vi "AlliGator Read RecSettings.txt File.vi"(8 "Error In":errorcluster, 11 "Folder Path":path) -> (0 "Error Out":errorcluster, 1 "Metadata":T1 {"Date" format="%<%x %.3X>T"}, 3 "Settings String":string)   [LabVIEW 2021, in "AlliGator Files.lvlib"]
doc: "Tries to extract FLI dataset metadata corresponding to one of LaVision formats."
uses:
  AlliGator Files.lvlib
  AlliGator RecSettings Metadata.ctl
  AlliGator RecSettings Metadata Field.ctl
  <vilib>/Utility/error.llb/whitespace.ctl
  Time/PicoStart Date.ctl
  <vilib>/Utility/error.llb/Error Cluster From Error Code.vi
  <vilib>/ErrorRing/Error Ring.xnode
  Time/Time.lvlib
  Error/Error.lvlib
panel:
  # "see the AlliGator License on the block diagram (Ctrl+E or Window:Show Block Diagram)"
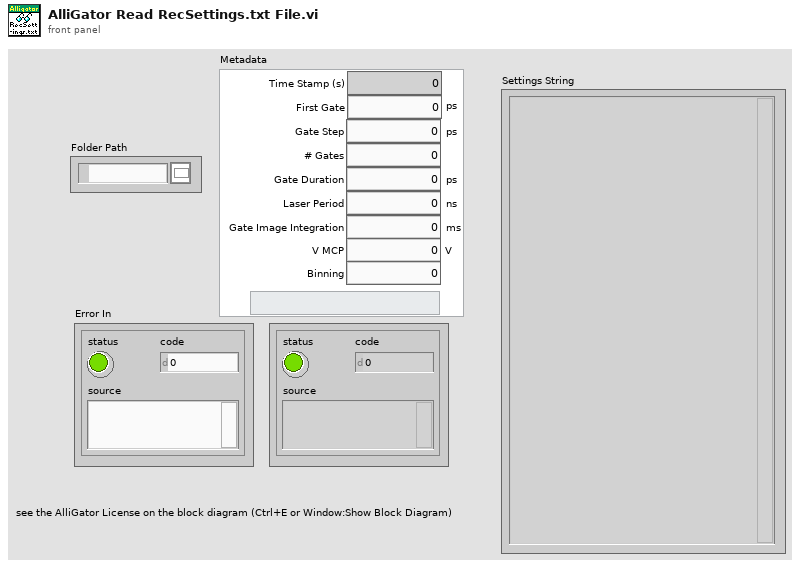
[diagram p1: front panel]
types:
  T1 = typedef "AlliGator Files.lvlib/AlliGator RecSettings Metadata.ctl" = cluster{"Time Stamp (s)":dbl, "First Gate":dbl[unit], "Gate Step":dbl[unit], "# Gates":i32, "Gate Duration":dbl[unit], "Laser Period":dbl[unit], "Gate Image Integration":dbl[unit], "Date":timestamp, "V MCP":dbl[unit], "Binning":dbl}
  T2 = typedef "Time.lvlib/PicoStart Date.ctl" = cluster{"Day in Week":string, "Month":string, "Day":i32, "Hours":i32, "Minutes":i32, "Seconds":i32, "Year":i32}
  T3 = typedef "AlliGator Files.lvlib/AlliGator RecSettings Metadata Field.ctl" = enum16{"Time", "Gate Start", "Gate Step", "# Gates", "Gate Duration", "Laser Period", "Gate Image Integration", "MCP Voltage", "Binning"}
  T4 = typedef "whitespace.ctl" = u16
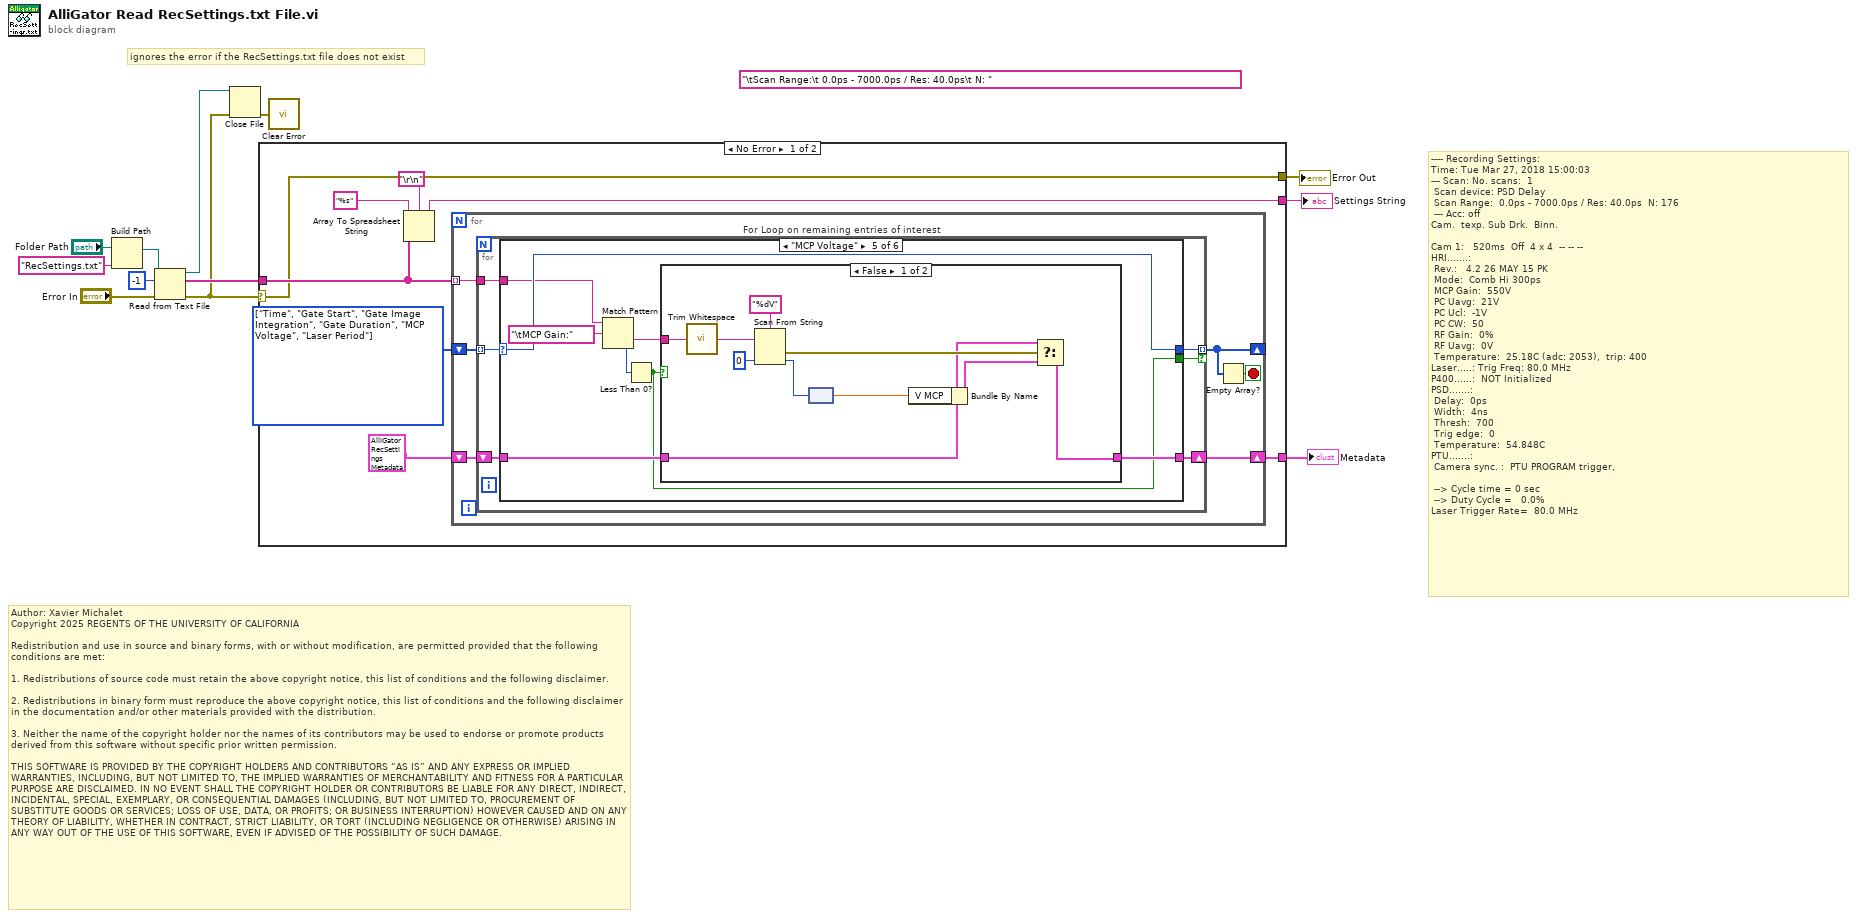
[diagram p0: block diagram]
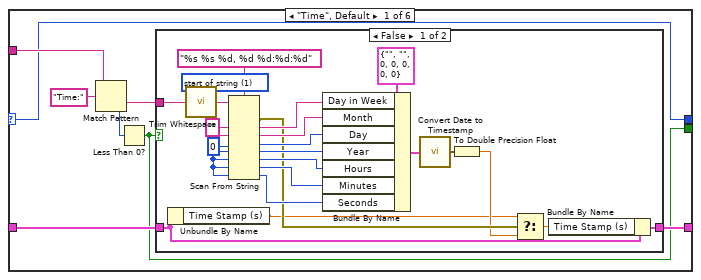
[diagram p2: hidden frame]
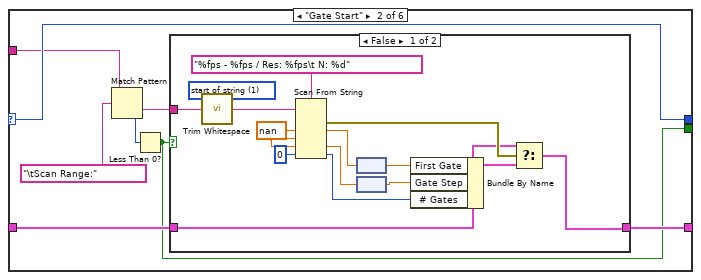
[diagram p4: hidden frame]
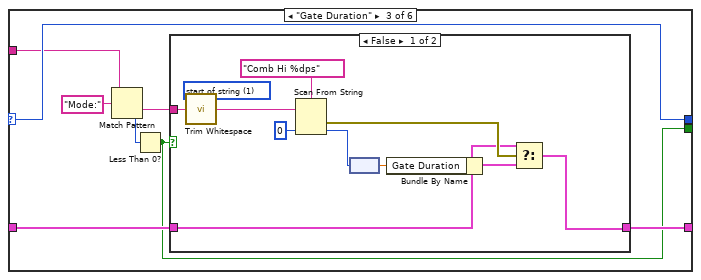
[diagram p6: hidden frame]
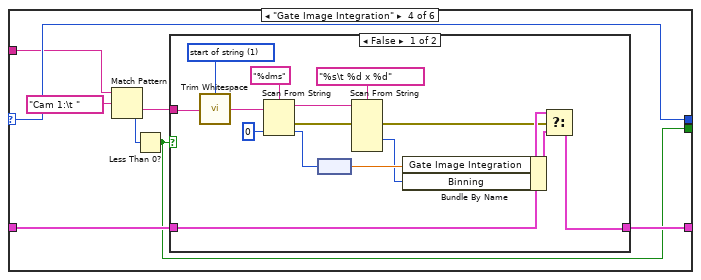
[diagram p8: hidden frame]
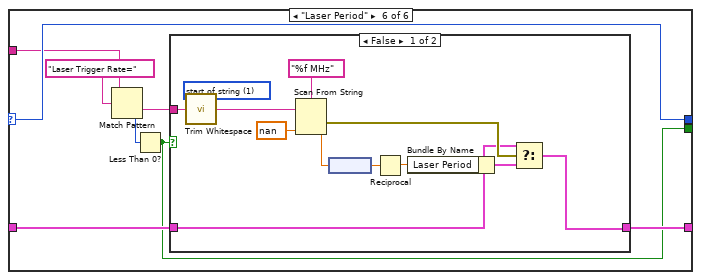
[diagram p11: hidden frame]
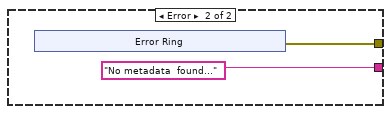
[diagram p13: hidden frame]
diagram:
  (unwired) "\tScan Range:\t 0.0ps - 7000.0ps / Res: 40.0ps\t N: "
  # "Author: Xavier Michalet\nCopyright 2025 REGENTS OF THE UNIVERSITY OF CALIFORNIA\n\nRedistribution and use in source and binary forms, with or without modification, are permitted provided that the following conditions are met:\n\n1. Redistributions of source code must retain the above copyright notice, this list of conditions and the following disclaimer.\n\n2. Redistributions in binary form must reproduce the above copyright notice, this list of conditions and the following disclaimer in the documentation and/or other materials provided with the distribution.\n\n3. Neither the name of the copyright holder nor the names of its contributors may be used to endorse or promote products derived from this software without specific prior written permission.\n\nTHIS SOFTWARE IS PROVIDED BY THE COPYRIGHT HOLDERS AND CONTRIBUTORS “AS IS” AND ANY EXPRESS OR IMPLIED WARRANTIES, INCLUDING, BUT NOT LIMITED TO, THE IMPLIED WARRANTIES OF MERCHANTABILITY AND FITNESS FOR A PARTICULAR PURPOSE ARE DISCLAIMED. IN NO EVENT SHALL THE COPYRIGHT HOLDER OR CONTRIBUTORS BE LIABLE FOR ANY DIRECT, INDIRECT, INCIDENTAL, SPECIAL, EXEMPLARY, OR CONSEQUENTIAL DAMAGES (INCLUDING, BUT NOT LIMITED TO, PROCUREMENT OF SUBSTITUTE GOODS OR SERVICES; LOSS OF USE, DATA, OR PROFITS; OR BUSINESS INTERRUPTION) HOWEVER CAUSED AND ON ANY THEORY OF LIABILITY, WHETHER IN CONTRACT, STRICT LIABILITY, OR TORT (INCLUDING NEGLIGENCE OR OTHERWISE) ARISING IN ANY WAY OUT OF THE USE OF THIS SOFTWARE, EVEN IF ADVISED OF THE POSSIBILITY OF SUCH DAMAGE."
  # "---- Recording Settings:\t\t\t\t\t\t\t\nTime:\tTue Mar 27, 2018 15:00:03\n--- Scan:\tNo. scans: \t1\n\tScan device:\tPSD Delay\n\tScan Range:\t 0.0ps - 7000.0ps / Res: 40.0ps\t N: 176\n\t--- Acc:\toff\nCam.\t texp.\tSub Drk. \tBinn.\n\nCam 1:\t  520ms\t Off\t 4 x 4\t\t--\t--\t--\nHRI.......:\n\tRev.: \t 4.2 26 MAY 15 PK \n\tMode: \tComb Hi 300ps\n\tMCP Gain: \t550V\n\tPC Uavg: \t21V\n\tPC Ucl: \t-1V\n\tPC CW: \t50\n\tRF Gain: \t0%\n\tRF Uavg: \t0V\n\tTemperature: \t25.18C (adc: 2053),  trip: 400\nLaser.....:\tTrig Freq: 80.0 MHz\nP400......:\t NOT Initialized\nPSD.......:\n\tDelay: \t0ps\n\tWidth: \t4ns\n\tThresh: \t700\n\tTrig edge: \t0\n\tTemperature: \t54.848C\nPTU.......:\n\tCamera sync. : \tPTU PROGRAM trigger, \n\t\n --> Cycle time =\t0 sec\n --> Duty Cycle = \t 0.0%\nLaser Trigger Rate= \t80.0 MHz"
  # "ignores the error if the RecSettings.txt file does not exist"
  n1 = Build Path(base path="Folder Path", name or relative path="RecSettings.txt") -> (appended path=w7:path)
  n2 = Read from Text File(file (use dialog)=w7, count=-1, error in="Error In") -> (refnum out=w11:refnum<file>, text=w10:string[], error out=w4:errorcluster)  [unwired: 1 in, 1 out]
  n3 = Close File(refnum=w11, error in=w4) -> (error out=w1:errorcluster)  [unwired: 1 out]
  n4 = case shown="No Error" w4 {
    selector: w4 -> [w14 _]
    tunnel: w10 -> [w17 _]
    tunnel: [w19 "No metadata  found..." ("spreadsheet string")] -> w9
    tunnel: [w15 _] -> w3
    tunnel: [w14 w172] -> w2
    frame No Error {
      w16 = T3[] [enum."Time", enum."Gate Start", enum."Gate Image Integration", enum."Gate Duration", enum."MCP Voltage", enum."Laser Period"] items=["Time", "Gate Start", "Gate Step", "# Gates", "Gate Duration", "Laser Period", "Gate Image Integration", "MCP Voltage", "Binning"] ("Array")
      n5 = Array To Spreadsheet String(delimiter (Tab)="\r\n", array=w17, 3:"%s" ("format string")) -> (spreadsheet string=w19:string)
      n6 = for {
        shift-right: [w24] -> w15
        shift-left: T1 {"Time Stamp (s)"=nan, "First Gate"=nan, "Gate Step"=nan, "# Gates"=0, "Gate Duration"=nan, "Laser Period"=nan, "Gate Image Integration"=nan, "Date"=timestamp(0 s since 1904-01-01), "V MCP"=nan, "Binning"=nan} ("Metadata") -> [w25]
        tunnel: w17 -> [w23] mode=indexing
        shift-right: [w22] -> _
        shift-left: w16 -> [w26]
        stop <- w21 stop-if-true
        n7 = for "For Loop on remaining entries of interest" {
          tunnel: w26 -> [w32] mode=indexing
          shift-right: [w30] -> w24
          shift-left: w25 -> [w31]
          tunnel: w23 -> [w29]
          tunnel: [w28] -> w22 mode=indexing if=w27
          n8 = case shown="\"MCP Voltage\"" w32 {
            selector: w32 -> [w34 w66 w90 w110 w134 w153]
            tunnel: w31 -> [w37 w68 w92 w112 w136 w155]
            tunnel: [w36 w67 w91 w111 w135 w154] -> w30
            tunnel: w29 -> [w35 w64 w88 w108 w132 w151]
            tunnel: [w34 w66 w90 w110 w134 w153] -> w28
            tunnel: [w33 w65 w89 w109 w133 w152] -> w27
            frame "Time", Default {
              n9 = Match Pattern(string=w35, regular expression="Time:") -> (after substring=w38:string, offset past match=w39:i32)  [unwired: 1 in, 2 out]
              n10 = Less Than 0?(x=w39) -> (x < 0?=w33:bool)
              n11 = case shown="False" w33 {
                tunnel: w38 -> [w61 _]
                tunnel: w37 -> [w43 w63]
                tunnel: [w41 w63] -> w36
                frame False {
                  w45 = 0 ("default value 3")
                  w46 = "" ("default value 1")
                  w60 = T4 1 items=["both", "start of string", "end of string"] ("location (both)")
                  n12 = Unbundle By Name(w43) -> ("Time Stamp (s)"=w44:dbl)
                  n13 = call <vilib>:"Trim Whitespace.vi"("string"=w61, "location (both)"=w60) -> ("trimmed string"=w50:string)
                  n14 = Scan From String(format string="%s %s %d, %d %d:%d:%d", input string=w50, default 1=w46, default 2=w46, default 3=w45, default 4=w45, default 5=w45, default 6=w45, default 7=w45) -> (error out=w48:errorcluster, output 1=w59:string, output 2=w58:string, output 3=w57:i32, output 4=w56:i32, output 5=w55:i32, output 6=w54:i32, output 7=w53:i32)  [unwired: 2 in, 2 out]
                  n15 = Bundle By Name(cluster=T2 {"Day in Week"="", "Month"="", "Day"=0, "Hours"=0, "Minutes"=0, "Seconds"=0, "Year"=0}, "Day in Week"=w59, "Month"=w58, "Day"=w57, "Year"=w56, "Hours"=w55, "Minutes"=w54, "Seconds"=w53) -> (w52:T2)
                  n16 = call "Convert Date to Timestamp.vi"("Date"=w52) -> ("Time Stamp"=w62:timestamp)  [unwired: 8 in]
                  n17 = To Double Precision Float(number=w62) -> (double precision float=w47:dbl)
                  n18 = Select(t=w44, s=w48, f=w47) -> (s? t:f=w42:dbl)
                  n19 = Bundle By Name(cluster=w43, "Time Stamp (s)"=w42) -> (w41:T1)
                }
                frame True {
                }
              }
            }
            frame "Gate Start" {
              n20 = Match Pattern(string=w64, regular expression="\tScan Range:") -> (after substring=w69:string, offset past match=w70:i32)  [unwired: 1 in, 2 out]
              n21 = Less Than 0?(x=w70) -> (x < 0?=w65:bool)
              n22 = case shown="False" w65 {
                tunnel: w69 -> [w76 _]
                tunnel: w68 -> [w79 w87]
                tunnel: [w77 w87] -> w67
                frame False {
                  w73 = nan ("default value 1")
                  w74 = T4 1 items=["both", "start of string", "end of string"] ("location (both)")
                  n23 = call <vilib>:"Trim Whitespace.vi"("string"=w76, "location (both)"=w74) -> ("trimmed string"=w75:string)
                  n24 = Scan From String(format string="%fps - %fps / Res: %fps\t N: %d", input string=w75, default 1=w73, default 2=w73, default 3=w73, default 4=0 ("default value 4")) -> (error out=w85:errorcluster, output 1=w84:dbl, output 3=w82:dbl, output 4=w80:i32)  [unwired: 3 in, 2 out]
                  n25 = node(w84) -> (w83:dbl[unit])
                  n26 = node(w82) -> (w81:dbl[unit])
                  n27 = Bundle By Name(cluster=w79, "First Gate"=w83, "Gate Step"=w81, "# Gates"=w80) -> (w78:T1)
                  n28 = Select(t=w79, s=w85, f=w78) -> (s? t:f=w77:T1)
                }
                frame True {
                }
              }
            }
            frame "Gate Duration" {
              n29 = Match Pattern(string=w88, regular expression="Mode:") -> (after substring=w93:string, offset past match=w94:i32)  [unwired: 1 in, 2 out]
              n30 = Less Than 0?(x=w94) -> (x < 0?=w89:bool)
              n31 = case shown="False" w89 {
                tunnel: w93 -> [w106 _]
                tunnel: w92 -> [w100 w107]
                tunnel: [w98 w107] -> w91
                frame False {
                  w97 = T4 1 items=["both", "start of string", "end of string"] ("location (both)")
                  n32 = call <vilib>:"Trim Whitespace.vi"("string"=w106, "location (both)"=w97) -> ("trimmed string"=w105:string)
                  n33 = Scan From String(format string="Comb Hi %dps", input string=w105, default 1=0 ("default value 1")) -> (error out=w103:errorcluster, output 1=w102:i32)  [unwired: 2 in, 2 out]
                  n34 = node(w102) -> (w101:dbl[unit])
                  n35 = Bundle By Name(cluster=w100, "Gate Duration"=w101) -> (w99:T1)
                  n36 = Select(t=w100, s=w103, f=w99) -> (s? t:f=w98:T1)
                }
                frame True {
                }
              }
            }
            frame "Gate Image Integration" {
              n37 = Match Pattern(string=w108, regular expression="Cam 1:\t ") -> (after substring=w113:string, offset past match=w114:i32)  [unwired: 1 in, 2 out]
              n38 = Less Than 0?(x=w114) -> (x < 0?=w109:bool)
              n39 = case shown="False" w109 {
                tunnel: w113 -> [w120 _]
                tunnel: w112 -> [w127 w131]
                tunnel: [w125 w131] -> w111
                frame False {
                  w118 = T4 1 items=["both", "start of string", "end of string"] ("location (both)")
                  n40 = call <vilib>:"Trim Whitespace.vi"("string"=w120, "location (both)"=w118) -> ("trimmed string"=w119:string)
                  n41 = Scan From String(format string="%dms", input string=w119, default 1=0 ("default value 1")) -> (remaining string=w123:string, error out=w122:errorcluster, output 1=w129:i32)  [unwired: 2 in, 1 out]
                  n42 = node(w129) -> (w128:dbl[unit])
                  n43 = Scan From String(format string="%s\t %d x %d", input string=w123, error in=w122) -> (error out=w121:errorcluster, output 2=w116:i32)  [unwired: 6 in, 2 out]
                  n44 = Bundle By Name(cluster=w127, "Gate Image Integration"=w128, "Binning"=w116) -> (w126:T1)
                  n45 = Select(t=w127, s=w121, f=w126) -> (s? t:f=w125:T1)
                }
                frame True {
                }
              }
            }
            frame "MCP Voltage" {
              n46 = Match Pattern(string=w132, regular expression="\tMCP Gain:") -> (after substring=w137:string, offset past match=w138:i32)  [unwired: 1 in, 2 out]
              n47 = Less Than 0?(x=w138) -> (x < 0?=w133:bool)
              n48 = case shown="False" w133 {
                tunnel: w137 -> [w141 _]
                tunnel: w136 -> [w145 w150]
                tunnel: [w143 w150] -> w135
                frame False {
                  n49 = call <vilib>:"Trim Whitespace.vi"("string"=w141) -> ("trimmed string"=w140:string)  [unwired: 1 in]
                  n50 = Scan From String(format string="%dV", input string=w140, default 1=0 ("default value 1")) -> (error out=w148:errorcluster, output 1=w147:i32)  [unwired: 2 in, 2 out]
                  n51 = node(w147) -> (w146:dbl[unit])
                  n52 = Bundle By Name(cluster=w145, "V MCP"=w146) -> (w144:T1)
                  n53 = Select(t=w145, s=w148, f=w144) -> (s? t:f=w143:T1)
                }
                frame True {
                }
              }
            }
            frame "Laser Period" {
              n54 = Match Pattern(string=w151, regular expression="Laser Trigger Rate=") -> (after substring=w156:string, offset past match=w157:i32)  [unwired: 1 in, 2 out]
              n55 = Less Than 0?(x=w157) -> (x < 0?=w152:bool)
              n56 = case shown="False" w152 {
                tunnel: w156 -> [w170 _]
                tunnel: w155 -> [w164 w171]
                tunnel: [w162 w171] -> w154
                frame False {
                  w161 = T4 1 items=["both", "start of string", "end of string"] ("location (both)")
                  n57 = call <vilib>:"Trim Whitespace.vi"("string"=w170, "location (both)"=w161) -> ("trimmed string"=w169:string)
                  n58 = Scan From String(format string="%f MHz", input string=w169, default 1=nan ("default value 1")) -> (error out=w167:errorcluster, output 1=w166:dbl)  [unwired: 2 in, 2 out]
                  n59 = node(w166) -> (w165:dbl[unit])
                  n60 = Reciprocal(x=w165) -> (1/x=w160:dbl[unit])
                  n61 = Bundle By Name(cluster=w164, "Laser Period"=w160) -> (w163:T1)
                  n62 = Select(t=w164, s=w167, f=w163) -> (s? t:f=w162:T1)
                }
                frame True {
                }
              }
            }
          }
        }
        n63 = Empty Array?(array=w22) -> (empty?=w21:bool)
      }
    }
    frame Error {
      n64 = xnode "Error Ring"() -> ("error out"=w172:errorcluster)
    }
  }
  "Settings String" <- w9
  "Error Out" <- w2
  "Metadata" <- w3
  n65 = call "Clear Error.vi"("Error In"=w1) -> ()  [unwired: 8 in, 1 out]
